vi "Empty Acquired Data.vi"() -> (0 "Empty Acquired Data":T1)   [LabVIEW 2021, in "Acquisition.lvlib"]
doc: "(inline VI) Return an empty Acquired Data value. Use in-place of a block diagram constant.\n\nA cluster with all the data acquired by the application for a single timer-tick."
uses:
  Acquisition.lvlib
  Acquired Data.ctl
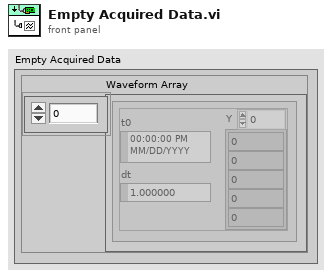
[diagram p1: front panel]
types:
  T1 = typedef "Acquisition.lvlib/Acquired Data.ctl" = cluster{"Waveform Array":waveform(dbl)[]}
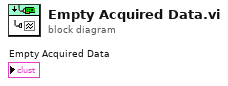
[diagram p0: block diagram]
diagram:
